vi "Shoot.vi"(10 "Duration":dbl) -> ()   [LabVIEW 2013]
uses:
  <vilib>/Rock Robotics/WPI/Solenoid/WPI_SolenoidValue.ctl
  Robot Global Data.vi
  Device Refrences.vi
  <vilib>/Rock Robotics/WPI/Solenoid/WPI_SolenoidSetEnum.vi
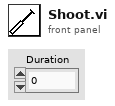
[diagram p1: front panel]
types:
  T1 = typedef "WPI_SolenoidValue.ctl" = enum16{"Off", "On", "Forward", "Reverse"}
  T2 = cluster{"Drive Output Values":dbl[], "Shooter Solenoid":T1, "Pickup Solenoid":T1}
  T3 = enum16{"Simulator Robot", "Alpinista", "2014 Robot"}
  T4 = typedef "WPI_SolenoidDevRef.ctl" = cluster{"DevStatus":errorcluster, "Solenoid Module":T5, "Forward Solenoid Channel":T6, "Reverse Solenoid Channel":T6}
  T5 = typedef "FPGA_TypedefSolenoidModule.ctl" = enum16{"Solenoid Module 1", "Solenoid Module 2"}
  T6 = typedef "WPI_SolenoidChannel.ctl" = enum8{"Solenoid 1", "Solenoid 2", "Solenoid 3", "Solenoid 4", "Solenoid 5", "Solenoid 6", "Solenoid 7", "Solenoid 8", "Invalid"}
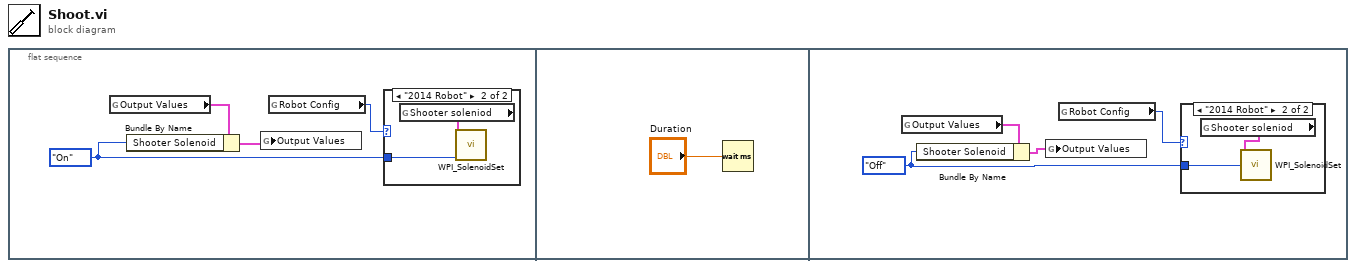
[diagram p0: block diagram]
diagram:
  n1 = flat-sequence {
    frame #0 {
      w3 = WPI_SolenoidValue."On" ("Value")
      n2 = global read "Robot Global Data.vi" "Output Values"() -> (w4:T2)
      n3 = Bundle By Name(cluster=w4, "Shooter Solenoid"=w3) -> (w2:T2)
      n4 = global write "Robot Global Data.vi" "Output Values"(w2) -> ()
      n5 = global read "Robot Global Data.vi" "Robot Config"() -> (w1:T3)
      n6 = case shown="\"2014 Robot\"" w1 {
        tunnel: w3 -> [_ w5]
        frame "Simulator Robot", Default {
        }
        frame "2014 Robot" {
          n7 = global read "Device Refrences.vi" "Shooter soleniod"() -> (w6:T4)
          n8 = call-poly <vilib>:"WPI_SolenoidSet.vi"("Value"=w5, "SolenoidDevRef"=w6) -> ()  [unwired: 8 in, 2 out]
        }
      }
    }
    frame #1 {
      n9 = Wait (ms)(milliseconds to wait="Duration") -> ()  [unwired: 1 out]
    }
    frame #2 {
      w10 = WPI_SolenoidValue."Off" ("Value")
      n10 = global read "Robot Global Data.vi" "Output Values"() -> (w9:T2)
      n11 = Bundle By Name(cluster=w9, "Shooter Solenoid"=w10) -> (w11:T2)
      n12 = global write "Robot Global Data.vi" "Output Values"(w11) -> ()
      n13 = global read "Robot Global Data.vi" "Robot Config"() -> (w8:T3)
      n14 = case shown="\"2014 Robot\"" w8 {
        tunnel: w10 -> [_ w13]
        frame "Simulator Robot", Default {
        }
        frame "2014 Robot" {
          n15 = global read "Device Refrences.vi" "Shooter soleniod"() -> (w12:T4)
          n16 = call-poly <vilib>:"WPI_SolenoidSet.vi"("Value"=w13, "SolenoidDevRef"=w12) -> ()  [unwired: 8 in, 2 out]
        }
      }
    }
  }
